vi "Create Order for X coordinate math.vi"(11 "Tree":T4) -> (3 "Array":T1[](array[typedef]))   [LabVIEW 2025]
uses:
  Types/Decision Tree.ctl
  Types/Sequencing Tree Node.ctl
  Types/Single Cmd Info.ctl
  <vilib>/picture/picture.llb/imagedata.ctl
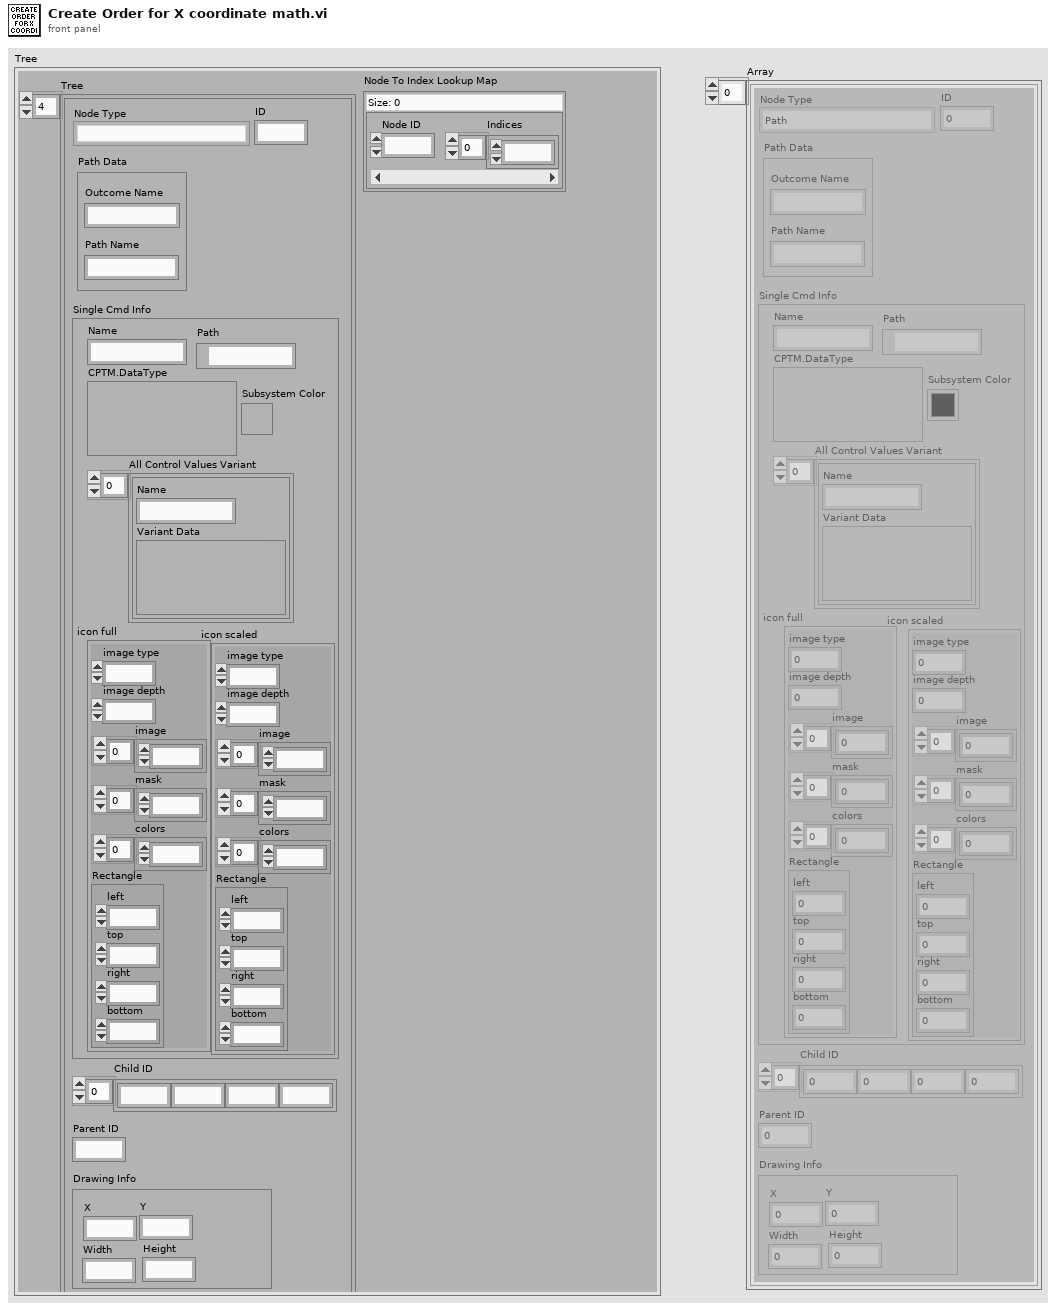
[diagram p1: front panel]
types:
  T1 = typedef "Sequencing Tree Node.ctl" = cluster{"Node Type":enum16{"Path", "Command", "Leaf"}, "ID":i16, "Path Data":cluster{"Path Name":string, "Outcome Name":string}, "Single Cmd Info":T2, "Child ID":i32[], "Parent ID":i32, "Drawing Info":cluster{"X":i32, "Y":i32, "Width":i32, "Height":i32}}
  T2 = typedef "Single Cmd Info.ctl" = cluster{"Name":string, "CPTM.DataType":variant, "All Control Values Variant":cluster{"Name":string, "Variant Data":variant}[], "icon full":T3, "icon scaled":T3, "Path":path, "Subsystem Color":u32}
  T3 = typedef "imagedata.ctl" = cluster{"image type":i32, "image depth":i32, "image":u8[], "mask":u8[], "colors":u32[], "Rectangle":cluster{"left":i16, "top":i16, "right":i16, "bottom":i16}}
  T4 = typedef "Decision Tree.ctl" = cluster{"Tree":T1[], "Node To Index Lookup Map":map{i16, i16[]}}
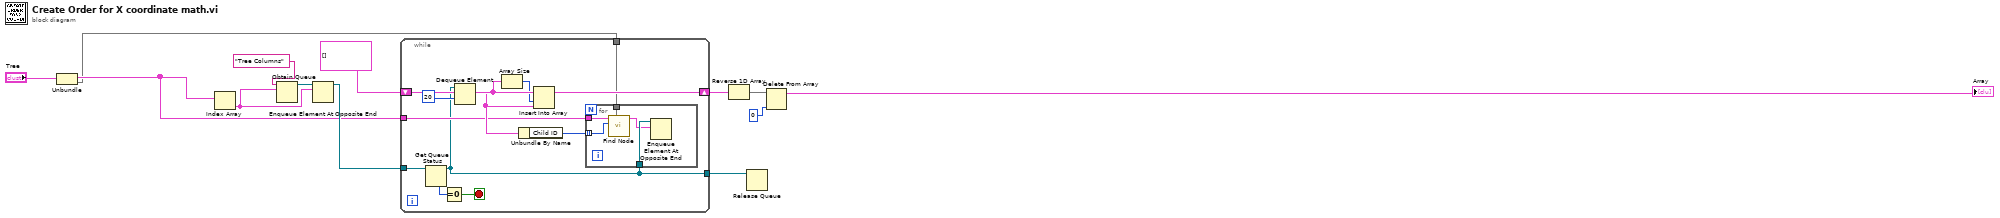
[diagram p0: block diagram]
diagram:
  n1 = Unbundle("Tree") -> ("Tree"=w2:T1[], "Node To Index Lookup Map"=w1:map{i16, i16[]})
  n2 = Index Array(array=w2) -> (element=w7:T1)  [unwired: 1 in]
  n3 = Obtain Queue(name (unnamed)="Tree Columns", element data type=w7) -> (queue out=w5:refnum<queue>)  [unwired: 3 in, 2 out]
  n4 = Enqueue Element At Opposite End(queue=w5, element=w7) -> (queue out=w6:refnum<queue>)  [unwired: 2 in, 2 out]
  n5 = while {
    tunnel: [w16] -> w8
    shift-right: [w19] -> w9
    shift-left: T1[] [] ("Sequencing Data 2") -> [w21]
    tunnel: w6 -> [w23]
    tunnel: w2 -> [w17]
    tunnel: w1 -> [w14]
    stop <- w25 stop-if-true
    n6 = Get Queue Status(queue=w23) -> (queue out=w16:refnum<queue>, # elements in queue=w24:i32)  [unwired: 2 in, 6 out]
    n7 = Equal To 0?(x=w24) -> (x = 0?=w25:bool)
    n8 = Dequeue Element(queue=w16, timeout in ms (-1)=20) -> (element=w18:T1)  [unwired: 1 in, 3 out]
    n9 = Array Size(array=w21) -> (size(s)=w20:i32)
    n10 = Unbundle By Name(w18) -> ("Child ID"=w15:i32[])
    n11 = Insert Into Array(array=w21, index=w20, new element=w18) -> (w19:T1[])
    n12 = for {
      tunnel: w15 -> [w27] mode=indexing
      tunnel: w17 -> [w28]
      tunnel: w16 -> [w30]
      tunnel: w14 -> [w26]
      n13 = call "Find Node.vi"("Node To Index Lookup Map"=w26, "ID"=w27, "Tree"=w28) -> ("Node"=w29:T1)  [unwired: 7 in, 1 out]
      n14 = Enqueue Element At Opposite End(queue=w30, element=w29) -> ()  [unwired: 2 in, 3 out]
    }
  }
  n15 = Reverse 1D Array(array=w9) -> (reversed array=w11:T1[])
  n16 = Release Queue(queue=w8) -> ()  [unwired: 2 in, 3 out]
  n17 = Delete From Array(array=w11, index=0) -> (array with subset deleted=→"Array":T1[])  [unwired: 1 in, 1 out]
